vi "Table-Equalise tables size.vi"(8 "error in (no error)":errorcluster, 9 "Tabe 2 (in)":string[][](array[string]), 11 "Table 1 (in)":string[][](array[string])) -> (0 "error out":errorcluster, 1 "Tabe 2":string[][](array[string]), 3 "Table 1":string[][](array[string]))   [LabVIEW 2020]
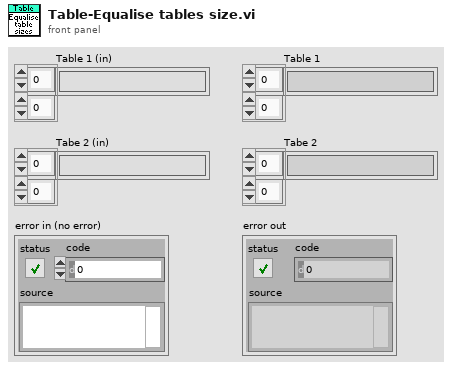
[diagram p1: front panel]
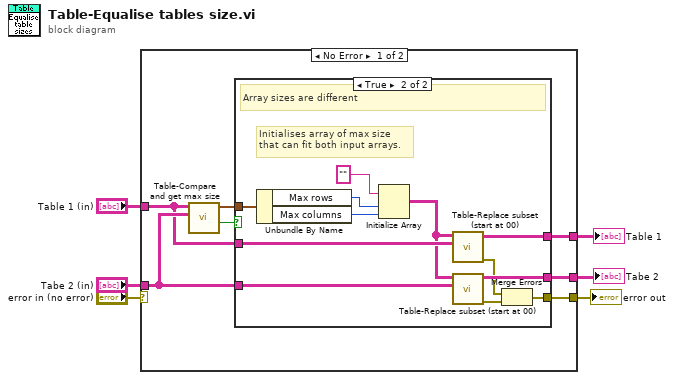
[diagram p0: block diagram]
diagram:
  n1 = case shown="No Error" "error in (no error)" {
    selector: "error in (no error)" -> [_ w30]
    tunnel: [w13 w28] -> w6
    tunnel: [w12 w29] -> w5
    tunnel: "Tabe 2 (in)" -> [w11 w28]
    tunnel: "Table 1 (in)" -> [w10 w29]
    tunnel: [w7 w30] -> w1
    frame No Error {
      n2 = call "Table-Compare and get max size.vi"("Table 2"=w11, "Table 1"=w10) -> ("Sizes are different"=w9:bool, "Max sizes"=w8:cluster{"Max rows":i32, "Max columns":i32})  [unwired: 8 in]
      n3 = case shown="True" w9 {
        tunnel: w8 -> [_ w27]
        tunnel: w10 -> [w15 w23]
        tunnel: w11 -> [w14 w22]
        tunnel: [w15 w20] -> w12
        tunnel: [w14 w19] -> w13
        tunnel: [_ w16] -> w7
        frame False {
        }
        frame True {
          # "Initialises array of max size \nthat can fit both input arrays."
          # "Array sizes are different"
          n4 = Unbundle By Name(w27) -> ("Max rows"=w26:i32, "Max columns"=w25:i32)
          n5 = Initialize Array("", w26, w25) -> (w21:string[][])
          n6 = call "Table-Replace subset (start at 00).vi"("Table to replace with"=w23, "Original table"=w21) -> ("error out"=w17:errorcluster, "Table out"=w20:string[][])  [unwired: 8 in]
          n7 = call "Table-Replace subset (start at 00).vi"("Table to replace with"=w22, "Original table"=w21) -> ("error out"=w18:errorcluster, "Table out"=w19:string[][])  [unwired: 8 in]
          n8 = Merge Errors(w17, w18) -> (w16:errorcluster)
        }
      }
    }
    frame Error {
    }
  }
  "Tabe 2" <- w6
  "Table 1" <- w5
  "error out" <- w1
